vi "komunikacja z GPS.vi"() -> ()   [LabVIEW 2012]
uses:
  <vilib>/robotics/Protocols/NMEA/typedefs/RMC Data.ctl
  <vilib>/robotics/Protocols/NMEA/typedefs/GGA Data.ctl
  <vilib>/robotics/Protocols/NMEA/typedefs/VTG Data.ctl
  <vilib>/robotics/Protocols/NMEA/typedefs/GSV Data.ctl
  <vilib>/robotics/Protocols/NMEA/typedefs/GLL Data.ctl
  <vilib>/robotics/Protocols/NMEA/typedefs/GSA Data.ctl
  <vilib>/Instr/_visa.llb/VISA Configure Serial Port (Instr).vi
  <vilib>/robotics/Protocols/NMEA/Advanced/Instrument Specific Poly VIs/GPS/Parse GLL Sentence.vi
  <vilib>/robotics/Protocols/NMEA/Advanced/Instrument Specific Poly VIs/GPS/Parse GSA Sentence.vi
  <vilib>/robotics/Protocols/NMEA/Advanced/Instrument Specific Poly VIs/GPS/Parse VTG Sentence.vi
  <vilib>/robotics/Protocols/NMEA/Advanced/Instrument Specific Poly VIs/GPS/Parse GSV Sentence.vi
  <vilib>/robotics/Protocols/NMEA/Advanced/Instrument Specific Poly VIs/GPS/Parse RMC Sentence.vi
  <vilib>/robotics/Protocols/NMEA/Advanced/Instrument Specific Poly VIs/GPS/Parse GGA Sentence.vi
  <vilib>/robotics/Protocols/NMEA/Advanced/Instrument Specific Poly VIs/GPS/Form GLL Sentence.vi
  <vilib>/robotics/Protocols/NMEA/Advanced/Instrument Specific Poly VIs/GPS/Form GSA Sentence.vi
  <vilib>/robotics/Protocols/NMEA/Advanced/Instrument Specific Poly VIs/GPS/Form VTG Sentence.vi
  <vilib>/robotics/Protocols/NMEA/Advanced/Instrument Specific Poly VIs/GPS/Form GSV Sentence.vi
  <vilib>/robotics/Protocols/NMEA/Advanced/Instrument Specific Poly VIs/GPS/Form GGA Sentence.vi
  <vilib>/robotics/Protocols/NMEA/NMEA API.lvlib
panel:
  out "GSA sentence":string
  out "GSA data":T1 {"type of fix"."mode" items=["", "No Fix", "2D Fix", "3D Fix"]; "selection of fix"."selection of 2D or 3D fix" items=["Automatic", "Manual"]}
  out "GLL sentence":string
  out "GLL data":T2 {"type of fix"."mode" items=["Simulator", "Not Valid", "Estimated", "Differential", "Autonomous"]; "status"."value" items=["Void", "Active"]; "time of fix"."time (UTC)" format="%^<%.3X\n%x>T"}
  out "GSV data":T3 {"satellite data"."data"."signal to noise ratio" min=0 max=99; "satellite data"."data"."azimuth (deg)" min=0 max=359; "satellite data"."data"."elevation (deg)" min=0 max=90; "number of satellites in view"."number of satellites" min=0; "sentence index"."index" min=0; "number of sentences for full data"."number of sentences" min=0}
  out "GSV sentence":string
  out "VTG  data":T4 {"type of fix"."mode" items=["Simulator", "Not Valid", "Estimated", "Differential", "Autonomous"]}
  out "VTG sentence":string
  out "concatenated string":string
  out "GGA sentence":string
  out "return count":u32
  out "GPRMC":string
  out "GGA data":T5 {"DGPS station ID number"."station ID number" min=0.0; "fix quality"."quality" items=["Invalid", "GPS Fix", "DGPS Fix", "PPS Fix", "Real Time Kinematic", "Float RTK", "Estimated", "Manual Input Mode", "Simulation Mode"]; "time of fix"."time (UTC)" format="%^<%.3X\n%x>T"}
  out "read buffer":string
  out "RMC data":T6={"time of fix"={"included?"=FALSE, "time (UTC)"=timestamp(1483228800 s since 1904-01-01)}, "status"={"included?"=FALSE, "value"=0}, "latitude"={"included?"=FALSE, "latitude (deg)"=0.0}, "longitude"={"included?"=FALSE, "longitude (deg)"=0.0}, "ground speed"={"included?"=FALSE, "speed (knots)"=0.0}, "true track angle"={"included?"=FALSE, "angle (deg)"=0.0}, "magnetic variation"={"included?"=FALSE, "variation (deg)"=0.0}, "type of fix"={"included?"=FALSE, "mode"=0}} {"type of fix"."mode" items=["Simulator", "Not Valid", "Estimated", "Differential", "Autonomous"]; "status"."value" items=["Void", "Active"]; "time of fix"."time (UTC)" format=" %^<%.3X\n%x>T"}
  in  "stop":bool
  in  "VISA resource name":refnum<visa-resource-name>
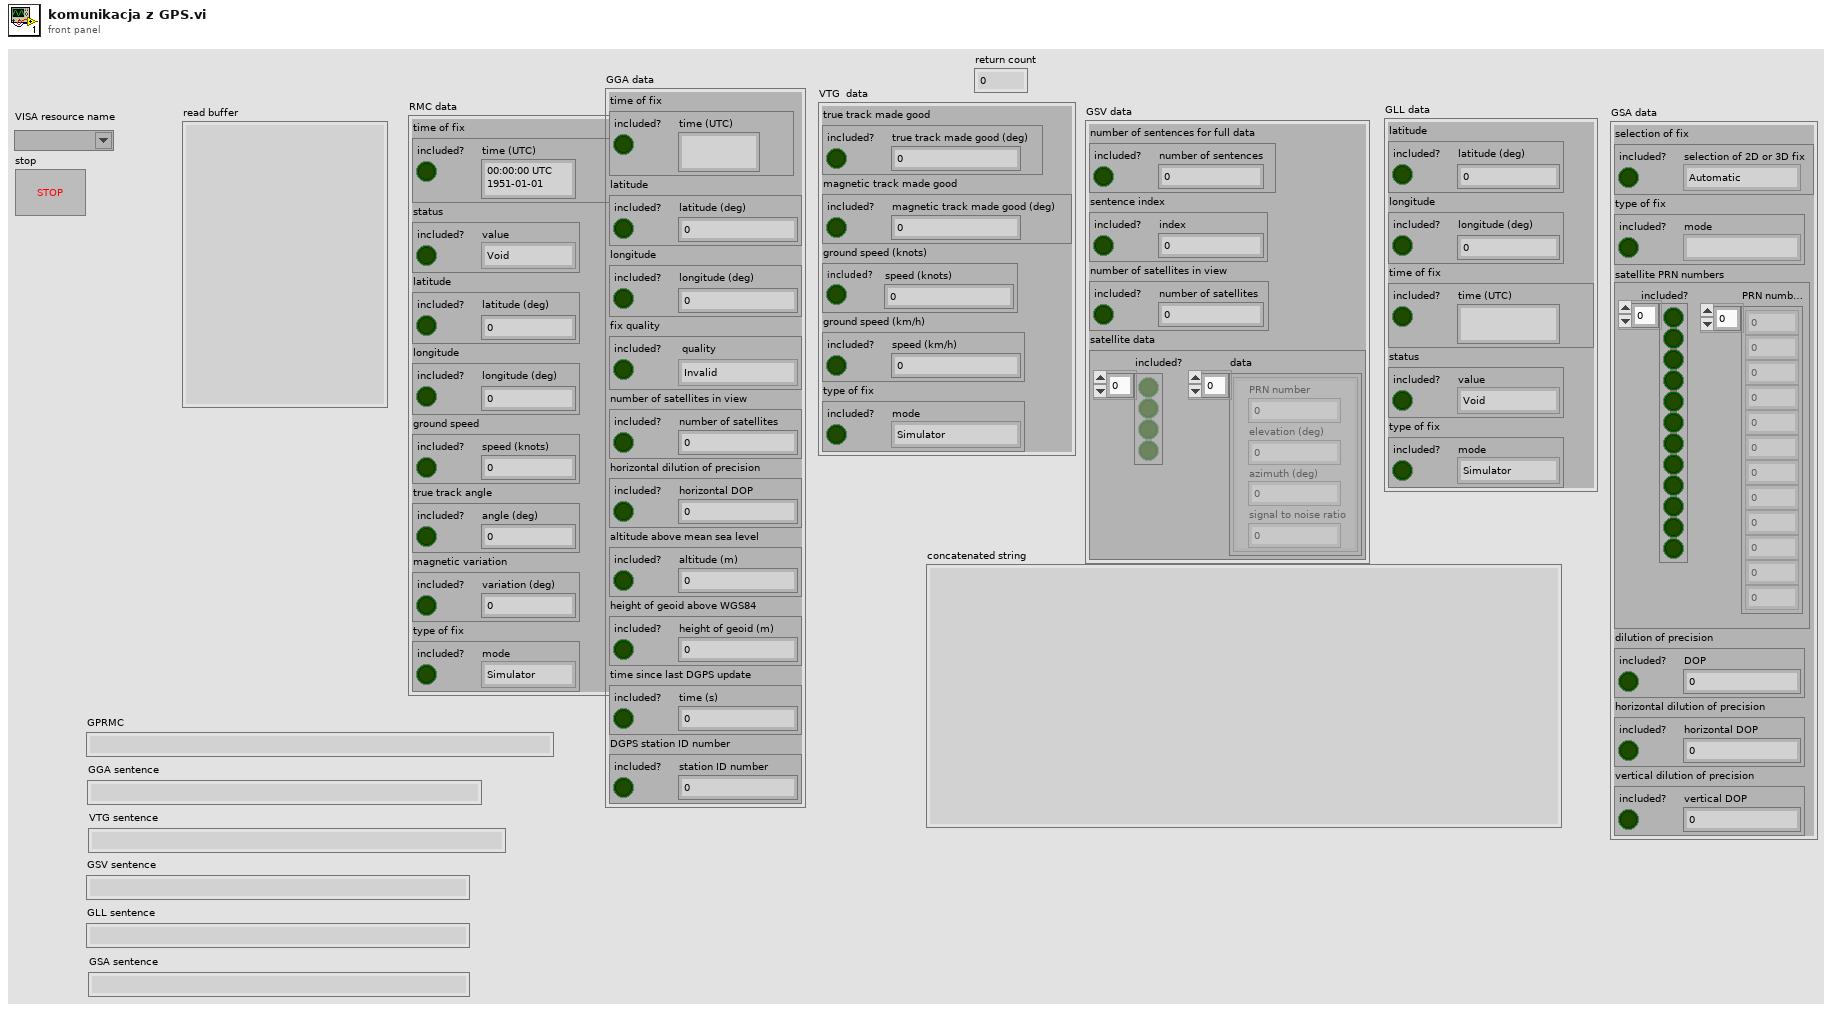
[diagram p1: front panel]
types:
  T1 = typedef "NMEA API.lvlib/GSA Data.ctl" = cluster{"selection of fix":cluster{"included?":bool, "selection of 2D or 3D fix":u16}, "type of fix":cluster{"included?":bool, "mode":u16}, "satellite PRN numbers":cluster{"included?":bool[], "PRN numbers":i32[]}, "dilution of precision":cluster{"included?":bool, "DOP":dbl}, "horizontal dilution of precision":cluster{"included?":bool, "horizontal DOP":dbl}, "vertical dilution of precision":cluster{"included?":bool, "vertical DOP":dbl}}
  T2 = typedef "NMEA API.lvlib/GLL Data.ctl" = cluster{"latitude":cluster{"included?":bool, "latitude (deg)":dbl}, "longitude":cluster{"included?":bool, "longitude (deg)":dbl}, "time of fix":cluster{"included?":bool, "time (UTC)":timestamp}, "status":cluster{"included?":bool, "value":u16}, "type of fix":cluster{"included?":bool, "mode":u16}}
  T3 = typedef "NMEA API.lvlib/GSV Data.ctl" = cluster{"number of sentences for full data":cluster{"included?":bool, "number of sentences":i8}, "sentence index":cluster{"included?":bool, "index":i8}, "number of satellites in view":cluster{"included?":bool, "number of satellites":i8}, "satellite data":cluster{"included?":bool[], "data":cluster{"PRN number":i32, "elevation (deg)":i32, "azimuth (deg)":i32, "signal to noise ratio":i32}[]}}
  T4 = typedef "NMEA API.lvlib/VTG Data.ctl" = cluster{"true track made good":cluster{"included?":bool, "true track made good (deg)":dbl}, "magnetic track made good":cluster{"included?":bool, "magnetic track made good (deg)":dbl}, "ground speed (knots)":cluster{"included?":bool, "speed (knots)":dbl}, "ground speed (km/h)":cluster{"included?":bool, "speed (km/h)":dbl}, "type of fix":cluster{"included?":bool, "mode":u16}}
  T5 = typedef "NMEA API.lvlib/GGA Data.ctl" = cluster{"time of fix":cluster{"included?":bool, "time (UTC)":timestamp}, "latitude":cluster{"included?":bool, "latitude (deg)":dbl}, "longitude":cluster{"included?":bool, "longitude (deg)":dbl}, "fix quality":cluster{"included?":bool, "quality":u16}, "number of satellites in view":cluster{"included?":bool, "number of satellites":i8}, "horizontal dilution of precision":cluster{"included?":bool, "horizontal DOP":dbl}, "altitude above mean sea level":cluster{"included?":bool, "altitude (m)":dbl}, "height of geoid above WGS84":cluster{"included?":bool, "height of geoid (m)":dbl}, "time since last DGPS update":cluster{"included?":bool, "time (s)":dbl}, "DGPS station ID number":cluster{"included?":bool, "station ID number":dbl}}
  T6 = typedef "NMEA API.lvlib/RMC Data.ctl" = cluster{"time of fix":cluster{"included?":bool, "time (UTC)":timestamp}, "status":cluster{"included?":bool, "value":u16}, "latitude":cluster{"included?":bool, "latitude (deg)":dbl}, "longitude":cluster{"included?":bool, "longitude (deg)":dbl}, "ground speed":cluster{"included?":bool, "speed (knots)":dbl}, "true track angle":cluster{"included?":bool, "angle (deg)":dbl}, "magnetic variation":cluster{"included?":bool, "variation (deg)":dbl}, "type of fix":cluster{"included?":bool, "mode":u16}}
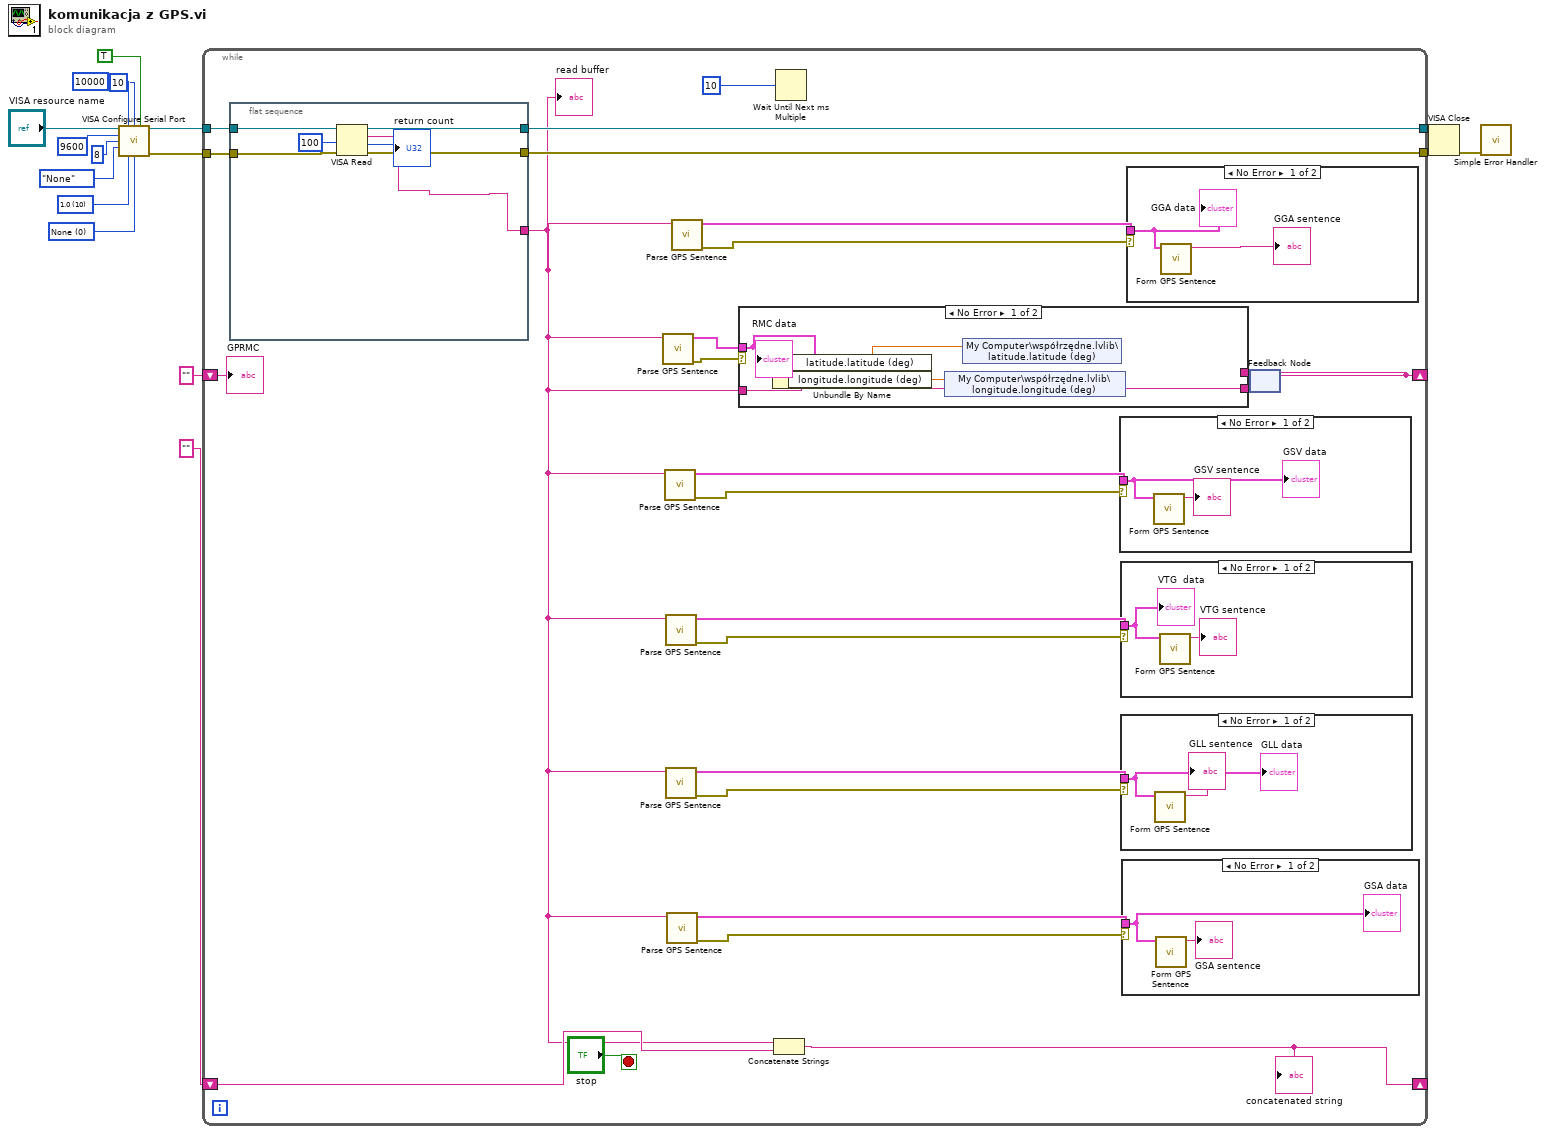
[diagram p0: block diagram]
diagram:
  w7 = u16 0 items=["None", "XON/XOFF", "RTS/CTS", "XON/XOFF & RTS/CTS", "DTR/DSR", "XON/XOFF & DTR/DSR"] ("flow control (0:none)")
  w8 = u16 10 items=["1.0"=10, "1.5"=15, "2.0"=20] ("stop bits (10: 1 bit)")
  n1 = call-poly "VISA Configure Serial Port"("VISA resource name"="VISA resource name", "timeout (10sec)"=u32 10000, "termination char\n(0xA = '\\n' = LF)"=u8 10 ("termination char\n(0xA = '\\n' = LF)"), "Enable Termination\nChar (T)"=TRUE ("Enable Termination\nChar (T)"), "baud rate (9600)"=u32 9600, "data bits (8)"=u16 8, "parity (0:none)"=enum16{"None", "Odd", "Even", "Mark", "Space"}."None", "stop bits (10: 1 bit)"=w8, "flow control (0:none)"=w7) -> ("VISA resource name out"=w12:refnum<visa-resource-name>, "error out"=w11:errorcluster)  [unwired: 5 in]
  n2 = while {
    tunnel: [w39] -> w5
    tunnel: [w38] -> w4
    tunnel: w12 -> [w37]
    tunnel: w11 -> [w36]
    shift-right: [w28] -> _
    shift-left: "" ("read buffer") -> [w30]
    shift-right: [w27] -> _
    shift-left: "" -> [w26]
    stop <- "stop" stop-if-true
    n3 = flat-sequence {
      tunnel: [w62] -> w39
      tunnel: [w61] -> w38
      tunnel: [w58] -> w17
      tunnel: w37 -> [w60]
      tunnel: w36 -> [w59]
      frame #0 {
        n4 = VISA Read(VISA resource name=w60, byte count=u32 100, error in (no error)=w59) -> (VISA resource name out=w62:refnum<visa-resource-name>, read buffer=w58:string, return count=→"return count":u32, error out=w61:errorcluster)
      }
    }
    n5 = call-poly <vilib>:"Parse GPS Sentence.vi"("RMC sentence"=w17) -> ("error out"=w34:errorcluster, "RMC data"=w33:T6)  [unwired: 9 in]
    n6 = call-poly <vilib>:"Parse GPS Sentence.vi"("GSV sentence"=w17) -> ("error out"=w25:errorcluster, "GSV data"=w24:T3)  [unwired: 9 in]
    n7 = call-poly <vilib>:"Parse GPS Sentence.vi"("VTG sentence"=w17) -> ("error out"=w22:errorcluster, "VTG  data"=w23:T4)  [unwired: 9 in]
    n8 = call-poly <vilib>:"Parse GPS Sentence.vi"("GLL sentence"=w17) -> ("error out"=w21:errorcluster, "GLL data"=w20:T2)  [unwired: 9 in]
    n9 = call-poly <vilib>:"Parse GPS Sentence.vi"("GSA sentence"=w17) -> ("error out"=w18:errorcluster, "GSA data"=w19:T1)  [unwired: 9 in]
    n10 = call-poly <vilib>:"Parse GPS Sentence.vi"("GGA sentence"=w17) -> ("error out"=w31:errorcluster, "GGA data"=w32:T5)  [unwired: 9 in]
    n11 = Concatenate Strings(w17, w26) -> (w27:string)
    "concatenated string" <- w27
    n12 = Wait Until Next ms Multiple(millisecond multiple=u32 10) -> ()  [unwired: 1 out]
    n13 = case shown="No Error" w25 {
      tunnel: w24 -> [w48 _]
      frame No Error {
        n14 = call-poly <vilib>:"Form GPS Sentence.vi"("GSV data"=w48) -> ("GSV sentence"=→"GSV sentence":string)  [unwired: 9 in, 1 out]
        "GSV data" <- w48
      }
      frame Error {
      }
    }
    n15 = case shown="No Error" w22 {
      tunnel: w23 -> [w46 _]
      frame No Error {
        n16 = call-poly <vilib>:"Form GPS Sentence.vi"("VTG  data"=w46) -> ("VTG sentence"=→"VTG sentence":string)  [unwired: 9 in, 1 out]
        "VTG  data" <- w46
      }
      frame Error {
      }
    }
    n17 = case shown="No Error" w21 {
      tunnel: w20 -> [w44 _]
      frame No Error {
        n18 = call-poly <vilib>:"Form GPS Sentence.vi"("GLL data"=w44) -> ("GLL sentence"=→"GLL sentence":string)  [unwired: 9 in, 1 out]
        "GLL data" <- w44
      }
      frame Error {
      }
    }
    n19 = case shown="No Error" w18 {
      tunnel: w19 -> [w42 _]
      frame No Error {
        n20 = call-poly <vilib>:"Form GPS Sentence.vi"("GSA data"=w42) -> ("GSA sentence"=→"GSA sentence":string)  [unwired: 9 in, 1 out]
        "GSA data" <- w42
      }
      frame Error {
      }
    }
    n21 = case shown="No Error" w31 {
      tunnel: w32 -> [w50 _]
      frame No Error {
        n22 = call-poly <vilib>:"Form GPS Sentence.vi"("GGA data"=w50) -> ("GGA sentence"=→"GGA sentence":string)  [unwired: 9 in, 1 out]
        "GGA data" <- w50
      }
      frame Error {
      }
    }
    n23 = feedback #1() -> (w28:string)  [unwired: 1 in]
    n24 = case shown="No Error" w34 {
      tunnel: w33 -> [w53 _]
      tunnel: w17 -> [w54 _]
      tunnel: [w54 w55] -> w29
      tunnel: w28 -> [_ w55]
      frame No Error {
        n25 = Unbundle By Name(w53) -> ("latitude.latitude (deg)"=w52:dbl, "longitude.longitude (deg)"=w51:dbl)
        n26 = shared-variable "My Computer\\współrzędne.lvlib\\longitude.longitude (deg)"(w51) -> ()  [unwired: 1 in, 1 out]
        n27 = shared-variable "My Computer\\współrzędne.lvlib\\latitude.latitude (deg)"(w52) -> ()  [unwired: 1 in, 1 out]
        "RMC data" <- w53
      }
      frame Error {
      }
    }
    n28 = feedback-in #1(w29) -> ()
    "read buffer" <- w17
    "GPRMC" <- w30
  }
  n29 = VISA Close(VISA resource name=w5, error in (no error)=w4) -> (error out=w15:errorcluster)
  n30 = call <vilib>:"Simple Error Handler.vi"("error in (no error)"=w15) -> ()  [unwired: 4 in, 5 out]
